vi "Destruct Tag_By Ref.vi"(8 "error in (no error)":errorcluster, 10 "Tag Ref in":refnum<data-value>) -> (0 "error out":errorcluster, 2 "deleted":bool)   [LabVIEW 2018, in "Tag Engine.lvlib" / "Tag Core.lvclass"]
doc: "Destruct a single CVT item by reference."
uses:
  Tag Core.lvclass
  Tag/Tag.lvclass
  Tag/Tag.lvclass/Tag.ctl
  Tag Core.lvclass/Tag Core.ctl
  Tag/Read Name.vi
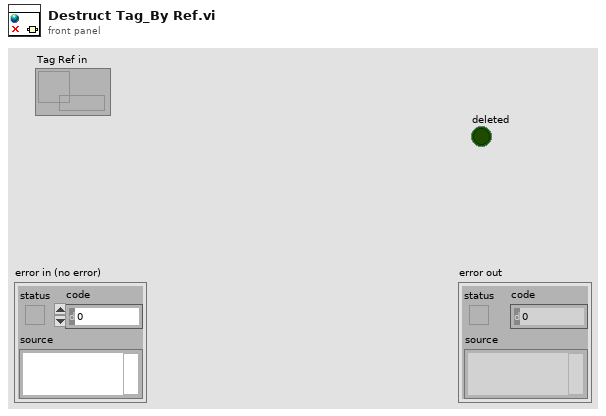
[diagram p1: front panel]
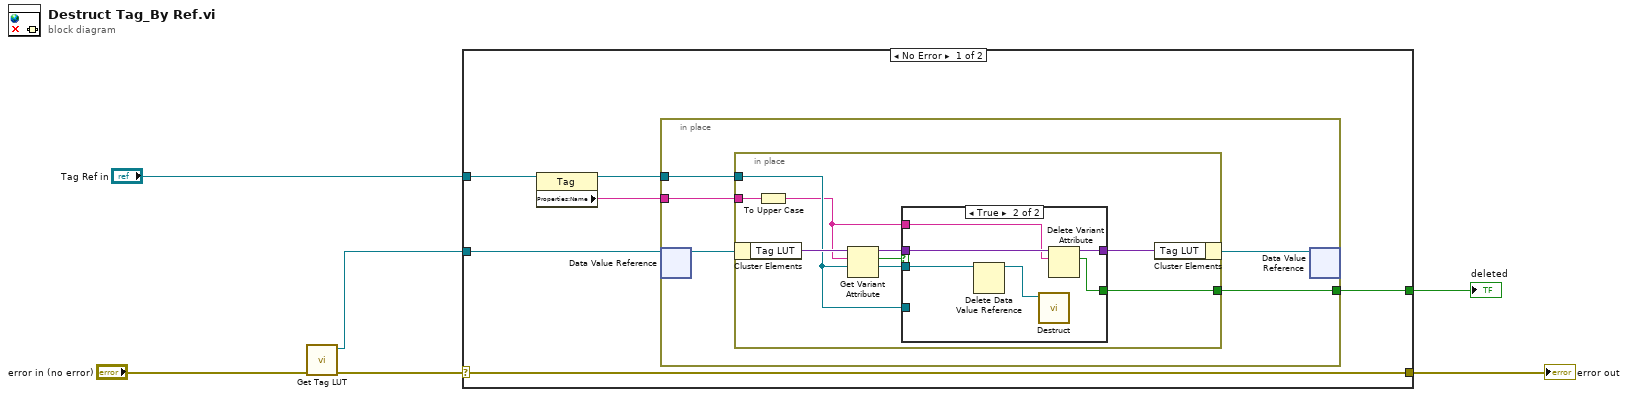
[diagram p0: block diagram]
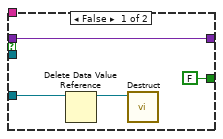
[diagram p2: hidden frame]
diagram:
  n1 = call "Get Tag LUT.vi"("error in (no error)"="error in (no error)") -> ("error out"=w4:errorcluster, "Tag LUT Out"=w3:refnum<data-value>)  [unwired: 9 in]
  n2 = case shown="No Error" w4 {
    selector: w4 -> [w12 w37]
    tunnel: [w12 w37] -> w6
    tunnel: w3 -> [w10 _]
    tunnel: "Tag Ref in" -> [w11 _]
    tunnel: [w7 _] -> w1
    frame No Error {
      n3 = property class="Tag"(reference=w11) -> (reference out=w8:refnum<data-value>, "Properties:Name"=w9:string)  [unwired: 1 in, 1 out]
      n4 = in-place {
        in-place-border: w9 -> [w16]
        in-place-border: w8 -> [w15]
        in-place-border: [w14] -> w7
        n5 = in-place-dvr #1(w10) -> (w17:refnum<class "Tag Core.lvclass">)  [unwired: 1 out]
        n6 = in-place {
          in-place-border: w16 -> [w19]
          in-place-border: w15 -> [w24]
          in-place-border: [w20] -> w14
          n7 = in-place-cluster #2(w17) -> ("Tag LUT"=w26:variant)
          n8 = To Upper Case(1:w19) -> (0:w18:string)
          n9 = Get Variant Attribute(Variant=w26, name=w18, default value (empty Variant)=w24) -> (duplicate Variant=w22:variant, found=w25:bool, value=w23:refnum<data-value>)  [unwired: 1 in, 1 out]
          n10 = case shown="True" w25 {
            tunnel: w24 -> [w29 _]
            tunnel: w23 -> [_ w36]
            tunnel: w22 -> [w30 w35]
            tunnel: w18 -> [_ w34]
            tunnel: [w30 w33] -> w21
            tunnel: [FALSE ("found") w32] -> w20
            frame False {
              n11 = Delete Data Value Reference(data value reference=w29) -> (data value=w27:refnum<class "Tag.lvclass">)  [unwired: 1 in, 1 out]
              n12 = call "Destruct.vi"("Tag in"=w27) -> ()  [unwired: 10 in, 1 out]
            }
            frame True {
              n13 = Delete Data Value Reference(data value reference=w36) -> (data value=w31:refnum<class "Tag.lvclass">)  [unwired: 1 in, 1 out]
              n14 = call "Destruct.vi"("Tag in"=w31) -> ()  [unwired: 10 in, 1 out]
              n15 = Delete Variant Attribute(6:w34, 7:w35) -> (2:w32:bool, 3:w33:variant)  [unwired: 1 in, 1 out]
            }
          }
          n16 = in-place-cluster #2("Tag LUT"=w21) -> (w13:refnum<class "Tag Core.lvclass">)
        }
        n17 = in-place-dvr #1(w13) -> ()  [unwired: 2 out]
      }
    }
    frame Error {
    }
  }
  "error out" <- w6
  "deleted" <- w1
